vi "Initialize Kalman Filter_avg_Magnetometer.vi"() -> (3 "Averaged Magnetometer-readings":T1)   [LabVIEW 2013]
uses:
  <vilib>/Analysis/Matrix/Datatypes/RealMatrix.ctl
  myRIO/Sensors/IMU/IMU_Data_Type_Def.ctl
  <vilib>/Analysis/Matrix/NI_Matrix.lvlib
panel:
  out "error out":errorcluster
  in  "error in (no error)":errorcluster
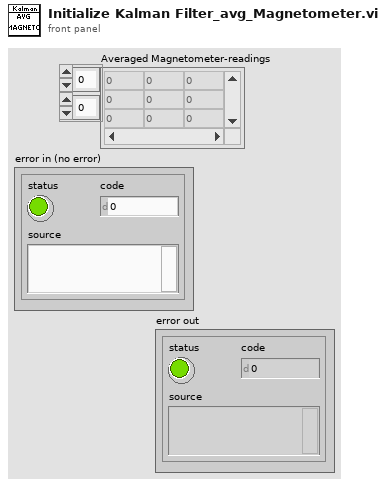
[diagram p1: front panel]
types:
  T1 = typedef "NI_Matrix.lvlib/RealMatrix.ctl" = dbl[][]
  T2 = typedef "IMU_Data_Type_Def.ctl" = cluster{timestamp, "X_Gyro_Out":dbl, "Y_Gyro_Out":dbl, "Z_Gyro_Out":dbl, "X_Accl_Out":dbl, "Y_Accl_Out":dbl, "Z_Accl_Out":dbl, "X_Magn_Out":dbl, "Y_Magn_Out":dbl, "Z_Magn_Out":dbl, "Temp_Out":dbl, "Barom_Out":dbl}
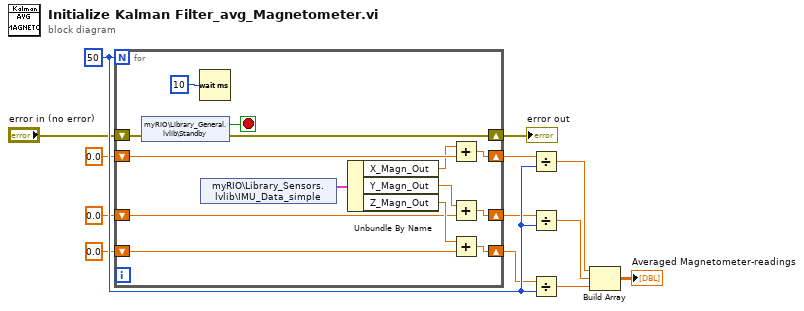
[diagram p0: block diagram]
diagram:
  w9 = 50
  n1 = for {
    N: w9 -> [_]
    shift-right: [w18] -> w6
    shift-left: 0.0 -> [w20]
    shift-right: [w21] -> w7
    shift-left: 0.0 -> [w23]
    shift-right: [w24] -> w8
    shift-left: 0.0 -> [w26]
    shift-right: [w14] -> w1
    shift-left: "error in (no error)" -> [w15]
    stop <- w16 stop-if-true
    n2 = shared-variable "myRIO\\Library_General.lvlib\\Standby"(error in=w15) -> (w16:bool, error out=w14:errorcluster)
    n3 = Wait (ms)(milliseconds to wait=u32 10) -> ()  [unwired: 1 out]
    n4 = shared-variable "myRIO\\Library_Sensors.lvlib\\IMU_Data_simple"() -> (w27:T2)  [unwired: 1 in, 1 out]
    n5 = Unbundle By Name(w27) -> ("X_Magn_Out"=w19:dbl, "Y_Magn_Out"=w22:dbl, "Z_Magn_Out"=w25:dbl)
    n6 = Add(x=w19, y=w20) -> (x+y=w18:dbl)
    n7 = Add(x=w22, y=w23) -> (x+y=w21:dbl)
    n8 = Add(x=w25, y=w26) -> (x+y=w24:dbl)
  }
  "error out" <- w1
  n9 = Divide(x=w6, y=w9) -> (x/y=w12:dbl)
  n10 = Divide(x=w7, y=w9) -> (x/y=w11:dbl)
  n11 = Divide(x=w8, y=w9) -> (x/y=w10:dbl)
  n12 = Build Array(w12, w11, w10) -> (→"Averaged Magnetometer-readings":T1)
